vi "Plot menu activation_.vi"(7 "menu tag":string, 8 "error in (no error)":errorcluster, 10 "MenuRef":refnum<k9>, 11 "BluePlotHandle in":refnum<class "RocketPlotHandle.lvclass">) -> (0 "error out":errorcluster, 2 "MenuRef":refnum<k9>, 3 "BluePlotHandle out":refnum<class "RocketPlotHandle.lvclass">)   [LabVIEW 2021, in "RocketPlotHandle.lvclass"]
uses:
  RocketPlotHandle.lvclass
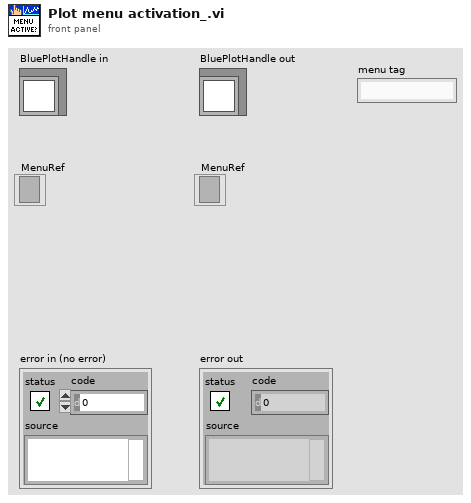
[diagram p1: front panel]
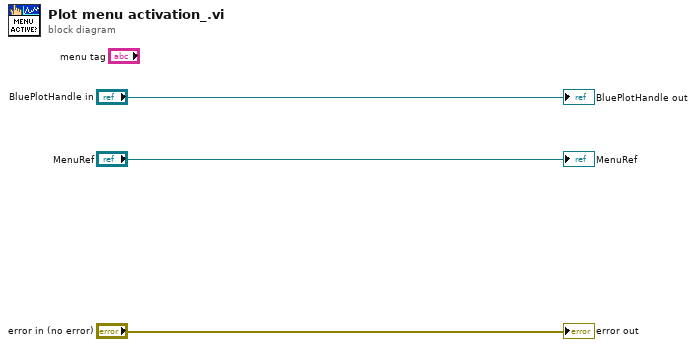
[diagram p0: block diagram]
diagram:
  "error out" <- "error in (no error)"
  "BluePlotHandle out" <- "BluePlotHandle in"
  "MenuRef" <- "MenuRef"
